vi "SendCommand.vi"(8 "error in (no error)":errorcluster, 11 "TCPComm in":refnum<class "TCPCommClass.lvclass">) -> (0 "error out":errorcluster, 3 "TCPComm out":refnum<class "TCPCommClass.lvclass">)   [LabVIEW 2013, in "TCPCommClass.lvclass"]
uses:
  TCPCommClass.lvclass
  TCPCommClass.lvclass/TCPCommClass.ctl
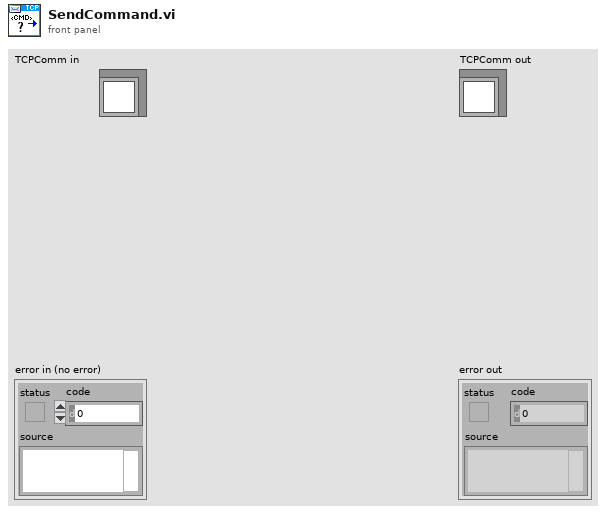
[diagram p1: front panel]
types:
  T1 = enum16{"Standard", "Buffered", "CRLF", "Immediate"}
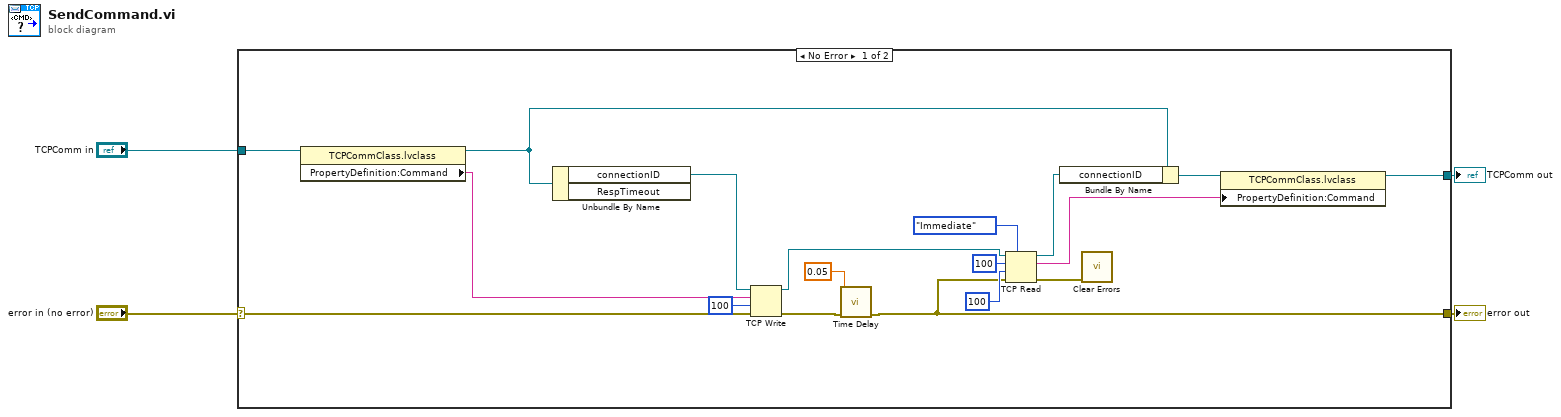
[diagram p0: block diagram]
diagram:
  n1 = case shown="No Error" "error in (no error)" {
    selector: "error in (no error)" -> [w22 w24]
    tunnel: [w5 w24] -> w3
    tunnel: [w15 w23] -> w1
    tunnel: "TCPComm in" -> [w20 w23]
    frame No Error {
      n2 = property class="TCPCommClass.lvclass"(reference=w20) -> (reference out=w19:refnum<class "TCPCommClass.lvclass">, "PropertyDefinition:Command"=w18:string)  [unwired: 1 in, 1 out]
      n3 = Unbundle By Name(w19) -> ("connectionID"=w21:refnum<k5>)  [unwired: 1 out]
      n4 = TCP Write(connection ID=w21, data in=w18, error in (no error)=w22, 9:100 ("bytes to read")) -> (connection ID out=w14:refnum<k5>, error out=w6:errorcluster)  [unwired: 1 out]
      n5 = call "Time Delay"("error in (no error)"=w6, "Delay Time (s)"=0.05) -> ("error out"=w5:errorcluster)  [unwired: 9 in]
      n6 = TCP Read(connection ID=w14, bytes to read=100, error in (no error)=w5, 7:T1."Immediate" ("mode (standard)"), 9:100 ("timeout ms (25000)")) -> (connection ID out=w13:refnum<k5>, data out=w9:string, error out=w10:errorcluster)
      n7 = Bundle By Name(cluster=w19, "connectionID"=w13) -> (w16:refnum<class "TCPCommClass.lvclass">)
      n8 = call <vilib>:"Clear Errors.vi"("error in (no error)"=w10) -> ()  [unwired: 6 in, 1 out]
      n9 = property class="TCPCommClass.lvclass"(reference=w16, "PropertyDefinition:Command"=w9) -> (reference out=w15:refnum<class "TCPCommClass.lvclass">)  [unwired: 1 in, 1 out]
    }
    frame Error {
    }
  }
  "error out" <- w3
  "TCPComm out" <- w1
